vi "Get Waveform Quadrature.vi"(8 "error in (no error)":errorcluster, 11 "Reference in":waveform(dbl)) -> (0 "error out":errorcluster, 2 "Reference Channel":string, 3 "Reference out":waveform(dbl))   [LabVIEW 2019, in "Lockin.DAQ.lvclass"]
uses:
  Lockin.DAQ.lvclass
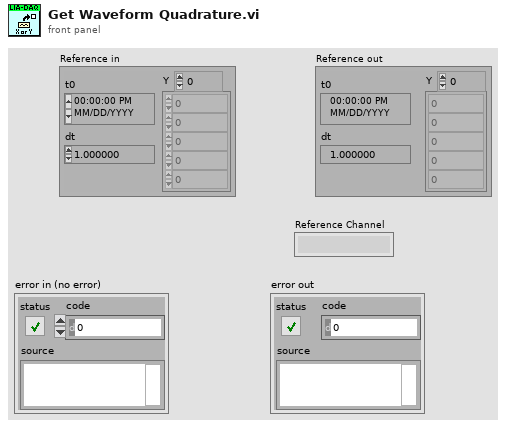
[diagram p1: front panel]
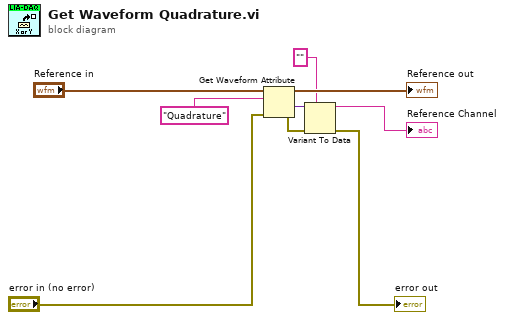
[diagram p0: block diagram]
diagram:
  n1 = Get Waveform Attribute(4:"error in (no error)", 6:"Quadrature" ("name"), 7:"Reference in") -> (0:w3:errorcluster, 1:w4:variant, 3:→"Reference out":waveform(dbl))  [unwired: 1 in, 1 out]
  n2 = Variant To Data(error in=w3, type="", Variant=w4) -> (data=→"Reference Channel":string, error out=→"error out":errorcluster)
